vi "Is Created Event.vi"(10 "Created Event Alias":string, 11 "qqqqq in":refnum<class "qqqqq.lvclass">) -> (2 "Is Created Event?":bool, 3 "qqqqq out":refnum<class "qqqqq.lvclass">)   [LabVIEW 2021, in "Providers.lvlib" / "qqqqq.lvlib" / "qqqqq.lvclass"]
uses:
  qqqqq.lvclass
  qqqqq.lvclass/qqqqq.ctl
  jettl/Queue/Queue.lvclass
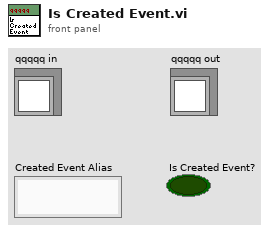
[diagram p1: front panel]
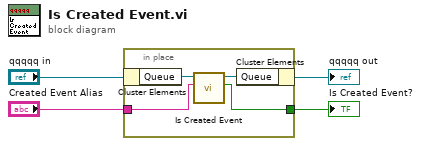
[diagram p0: block diagram]
diagram:
  n1 = in-place {
    in-place-border: [w6] -> w2
    in-place-border: "Created Event Alias" -> [w5]
    n2 = in-place-cluster #1("qqqqq in") -> ("Queue"=w8:refnum<class "Queue.lvclass">)
    n3 = call-dynamic "Is Created Event.vi"("Created Event Alias"=w5, "Queue in"=w8) -> ("Is Created Event?"=w6:bool, "Queue out"=w7:refnum<class "Queue.lvclass">)  [unwired: 8 in]
    n4 = in-place-cluster #1("Queue"=w7) -> (→"qqqqq out":refnum<class "qqqqq.lvclass">)
  }
  "Is Created Event?" <- w2
